vi "Send Settings.vi"(8 "error in (no error)":errorcluster, 11 "GEN40-38-LAN in":refnum<class "GEN40-38-LAN.lvclass">) -> (0 "error out":errorcluster, 3 "GEN40-38-LAN out":refnum<class "GEN40-38-LAN.lvclass">)   [LabVIEW 2018, in "GEN40-38-LAN.lvlib" / "GEN40-38-LAN.lvclass"]
uses:
  GEN40-38-LAN.lvclass
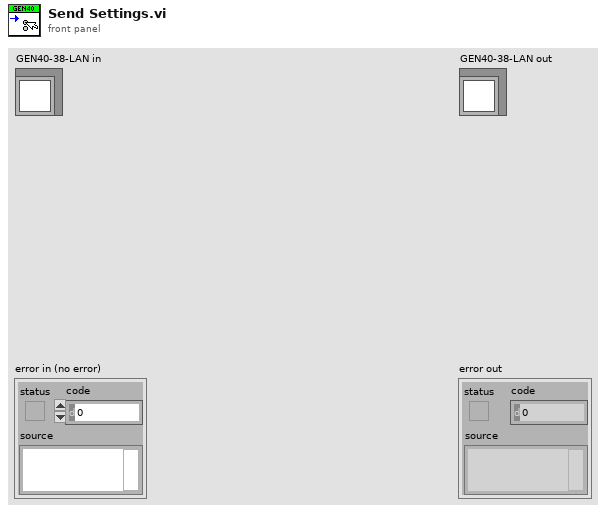
[diagram p1: front panel]
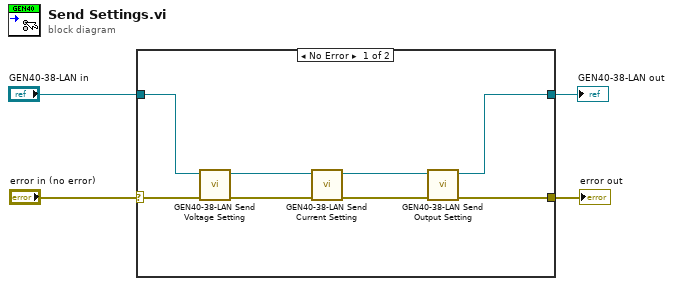
[diagram p0: block diagram]
diagram:
  n1 = case shown="No Error" "error in (no error)" {
    selector: "error in (no error)" -> [w12 w14]
    tunnel: [w6 w14] -> w3
    tunnel: [w7 w13] -> w2
    tunnel: "GEN40-38-LAN in" -> [w5 w13]
    frame No Error {
      n2 = call "GEN40-38-LAN Send Voltage Setting.vi"("error in (no error)"=w12, "GEN40-38-LAN in"=w5) -> ("error out"=w11:errorcluster, "GEN40-38-LAN out"=w10:refnum<class "GEN40-38-LAN.lvclass">)  [unwired: 8 in]
      n3 = call "GEN40-38-LAN Send Current Setting.vi"("error in (no error)"=w11, "GEN40-38-LAN in"=w10) -> ("error out"=w9:errorcluster, "GEN40-38-LAN out"=w8:refnum<class "GEN40-38-LAN.lvclass">)  [unwired: 8 in]
      n4 = call "GEN40-38-LAN Send Output Setting.vi"("error in (no error)"=w9, "GEN40-38-LAN in"=w8) -> ("error out"=w6:errorcluster, "GEN40-38-LAN out"=w7:refnum<class "GEN40-38-LAN.lvclass">)  [unwired: 8 in]
    }
    frame Error {
    }
  }
  "error out" <- w3
  "GEN40-38-LAN out" <- w2
